vi "Filter Data.vi"(8 "error in (no error)":errorcluster, 10 "Debug Data In":refnum<class "Debug Data.lvclass">[](array[class]), 11 "Filter by Process in":refnum<class "Filter by Is Action.lvclass">) -> (0 "error out":errorcluster, 2 "Debug Data Out":refnum<class "Debug Data.lvclass">[](array[class]), 3 "Filter by Process out":refnum<class "Filter by Is Action.lvclass">)   [LabVIEW 2020, in "Filter by Is Action.lvclass"]
uses:
  Filter by Is Action.lvclass
  Debug Data/Debug Data.lvclass
  Filter by Is Action.lvclass/Filter by Is Action.ctl
  Debug Data/Debug Data.lvclass/Debug Data.ctl
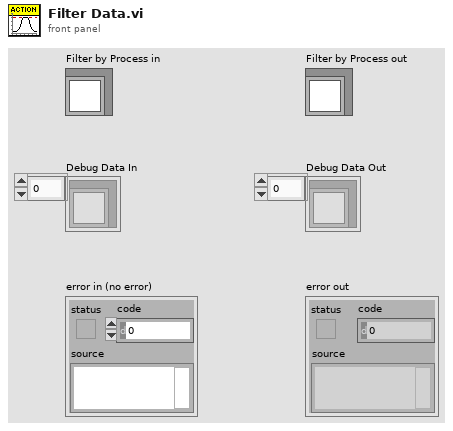
[diagram p1: front panel]
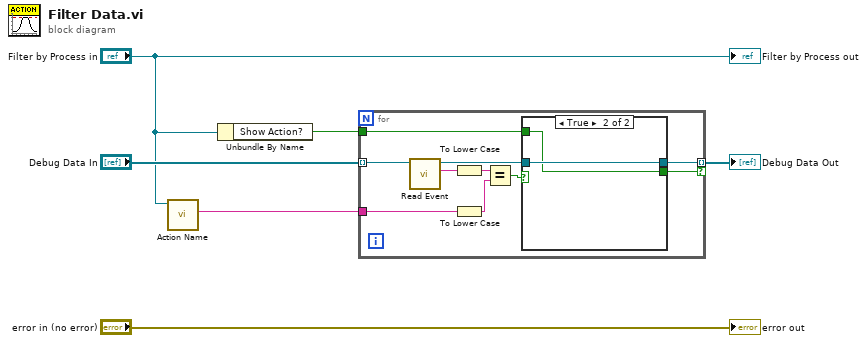
[diagram p0: block diagram]
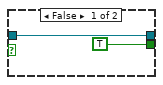
[diagram p2: hidden frame]
diagram:
  n1 = call-dynamic "Action Name.vi"("Filter by Is Action In"="Filter by Process in") -> ("Action Name"=w1:string)  [unwired: 8 in, 2 out]
  n2 = Unbundle By Name("Filter by Process in") -> ("Show Action?"=w3:bool)
  n3 = for {
    tunnel: [w14] -> w5 mode=indexing if=w12
    tunnel: "Debug Data In" -> [w16] mode=indexing
    tunnel: w3 -> [w11]
    tunnel: w1 -> [w9]
    n4 = call "Read Event.vi"("Debug Data in"=w16) -> ("Event"=w15:string, "Debug Data out"=w13:refnum<class "Debug Data.lvclass">)  [unwired: 9 in]
    n5 = To Lower Case(string=w15) -> (all lower case string=w10:string)
    n6 = To Lower Case(string=w9) -> (all lower case string=w7:string)
    n7 = Equal?(x=w10, y=w7) -> (x = y?=w8:bool)
    n8 = case shown="True" w8 {
      tunnel: [w18 w20] -> w14
      tunnel: w13 -> [w18 w20]
      tunnel: [TRUE ("Show Send?") w19] -> w12
      tunnel: w11 -> [_ w19]
      frame False {
      }
      frame True {
      }
    }
  }
  "Debug Data Out" <- w5
  "error out" <- "error in (no error)"
  "Filter by Process out" <- "Filter by Process in"
